vi "Init Events.vi"(8 "error in":errorcluster) -> (0 "error out":errorcluster, 3 "Request Events":T1)   [LabVIEW 2014, in "Chart Module.lvlib"]
uses:
  Chart Module.lvlib
  Request Events--cluster.ctl
  Stop Argument--cluster.ctl
  Show Panel Argument--cluster.ctl
  Hide Panel Argument--cluster.ctl
  Limits Argument--cluster.ctl
  Send Value Argument--cluster.ctl
  Clear Chart--arguments.ctl
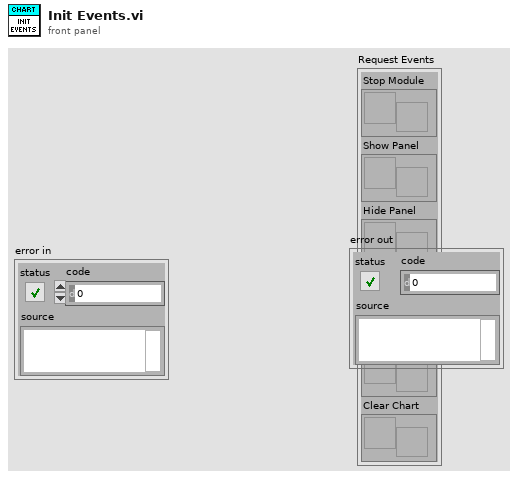
[diagram p1: front panel]
types:
  T1 = typedef "Chart Module.lvlib/Request Events--cluster.ctl" = cluster{"Stop Module":refnum<user-event>, "Show Panel":refnum<user-event>, "Hide Panel":refnum<user-event>, "Update Limits":refnum<user-event>, "Send Value":refnum<user-event>, "Clear Chart":refnum<user-event>}
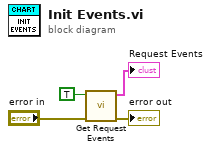
[diagram p0: block diagram]
diagram:
  n1 = call "Get Request Events.vi"("error in"="error in", "Create new?"=TRUE) -> ("error out"=→"error out":errorcluster, "Request Events"=→"Request Events":T1)  [unwired: 8 in]
